vi "NoteNode_Create.vi"(0 "reference":refnum<class "NoteNode.lvclass">, 5 "error in (no error)":errorcluster) -> (14 "reference out":refnum<class "NoteNode.lvclass">, 19 "error out":errorcluster)   [LabVIEW 2014, in "NoteNode.lvclass"]
doc: "Creates and initializes a new NoteNode object.\n\nThis object should be destroyed using a NoteNode destructor VI or a virtual base class destructor VI.\n\n[GOOP 2.1]"
uses:
  <resource>/Framework/Providers/Open_GDS/UML/NoteNode_class/NoteNode.lvclass
  <resource>/Framework/Providers/Open_GDS/UML/RectangularNode_class/RectangularNode.lvclass
  <resource>/Framework/Providers/Open_GDS/UML/MultiLineString_class/MultiLineString.lvclass
panel:
  # "The input reference should only\nbe wired when this method is called\nby a sub class constructor."
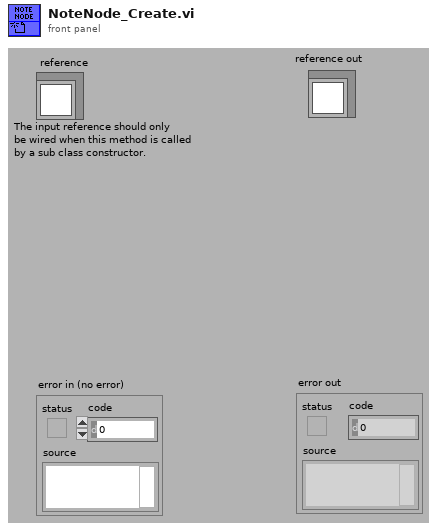
[diagram p1: front panel]
types:
  T1 = typedef "NoteNode.lvclass/ObjectAttributes.ctl" = cluster{"DEFAULT_WIDTH":i32, "DEFAULT_HEIGHT":i32, "DEFAULT_COLOR":u32, "FOLD_X":i32, "FOLD_Y":i32, "color":u32, "text":refnum<class "MultiLineString.lvclass">, "pointNodes":refnum<class "AbstractNode.lvclass">[]}
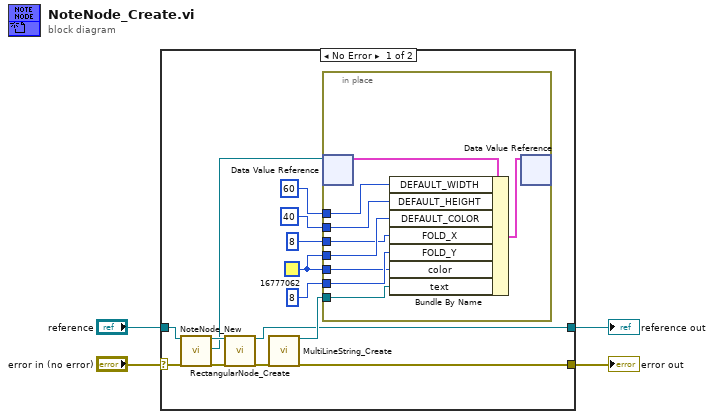
[diagram p0: block diagram]
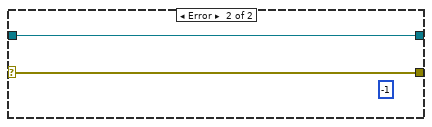
[diagram p2: hidden frame]
diagram:
  n1 = case shown="No Error" "error in (no error)" {
    selector: "error in (no error)" -> [w18 w29]
    tunnel: [w6 w28] -> w4
    tunnel: [w7 w29] -> w3
    tunnel: "reference" -> [w17 w28]
    frame No Error {
      w9 = u32 16777062
      n2 = call <resource>:"NoteNode_New.vi"("reference in"=w17, "error in (no error)"=w18) -> ("reference out"=w15:refnum<class "NoteNode.lvclass">, "DVRRefOut"=w5:refnum<data-value>, "error out"=w16:errorcluster)  [unwired: 2 in, 13 out]
      n3 = call <resource>:"RectangularNode_Create.vi"("reference"=w15, "error in (no error)"=w16) -> ("reference out"=w6:refnum<class "NoteNode.lvclass">, "error out"=w14:errorcluster)  [unwired: 1 in, 15 out]
      n4 = call <resource>:"MultiLineString_Create.vi"("error in (no error)"=w14) -> ("reference out"=w8:refnum<class "MultiLineString.lvclass">, "error out"=w7:errorcluster)  [unwired: 2 in, 15 out]
      n5 = in-place {
        in-place-border: 60 ("DEFAULT_WIDTH") -> [w26]
        in-place-border: 40 ("DEFAULT_HEIGHT") -> [w25]
        in-place-border: w9 -> [w24]
        in-place-border: 8 ("FOLD_X") -> [w23]
        in-place-border: 8 ("FOLD_Y") -> [w22]
        in-place-border: w9 -> [w21]
        in-place-border: w8 -> [w20]
        n6 = in-place-dvr #1(w5) -> (w27:T1)  [unwired: 1 out]
        n7 = Bundle By Name(cluster=w27, "DEFAULT_WIDTH"=w26, "DEFAULT_HEIGHT"=w25, "DEFAULT_COLOR"=w24, "FOLD_X"=w23, "FOLD_Y"=w22, "color"=w21, "text"=w20) -> (w19:T1)
        n8 = in-place-dvr #1(w19) -> ()  [unwired: 2 out]
      }
    }
    frame Error {
      (unwired) -1 ("Nr of open handles")
    }
  }
  "error out" <- w3
  "reference out" <- w4
